vi "Compare.vi"() -> ()   [LabVIEW 2013]
panel:
  out "Test":string
  in  "Use As Reference":bool
  in  "Next":bool
  in  "pattern":string="*.png"
  out "Reference Picture":picture
  out "Test Picture":picture
  in  "Reference Directory":path=path "C:/aplot/tests/ref"
  in  "Test Directory":path=path "C:/aplot/tests/output"
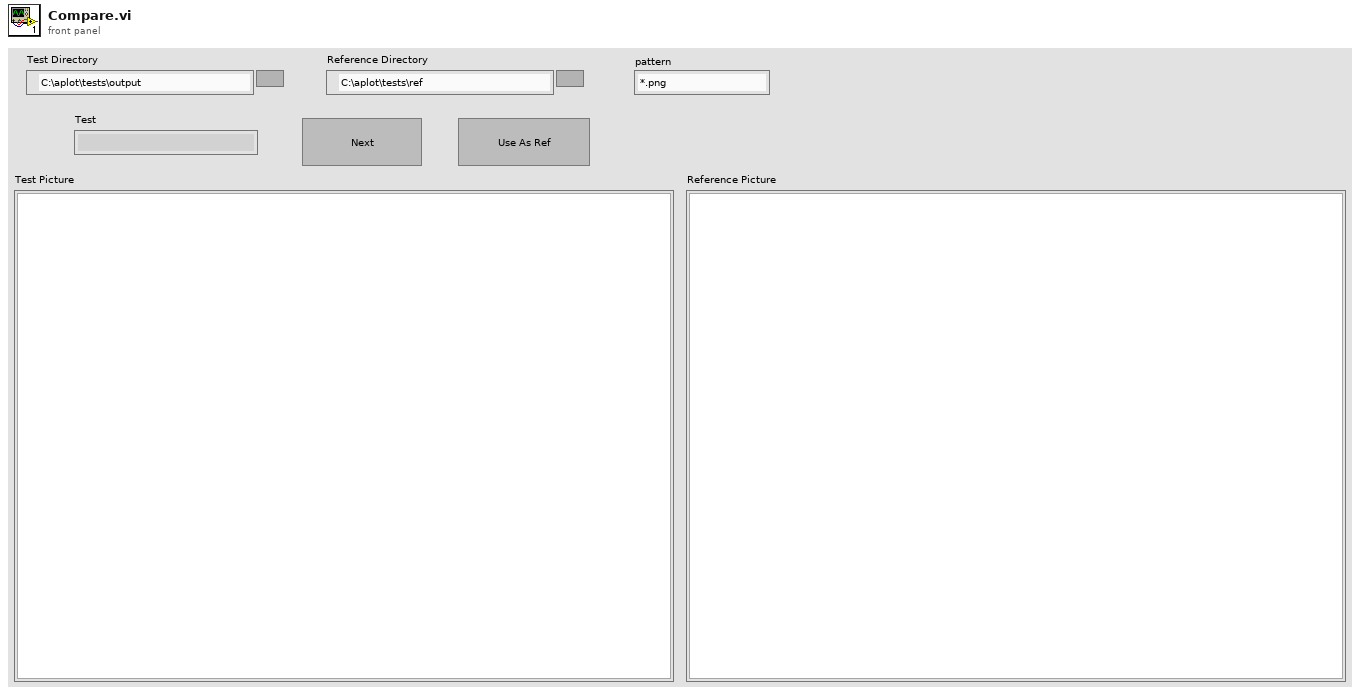
[diagram p1: front panel]
types:
  T1 = typedef "imagedata.ctl" = cluster{"image type":i32, "image depth":i32, "image":u8[], "mask":u8[], "colors":u32[], "Rectangle":cluster{"left":i16, "top":i16, "right":i16, "bottom":i16}}
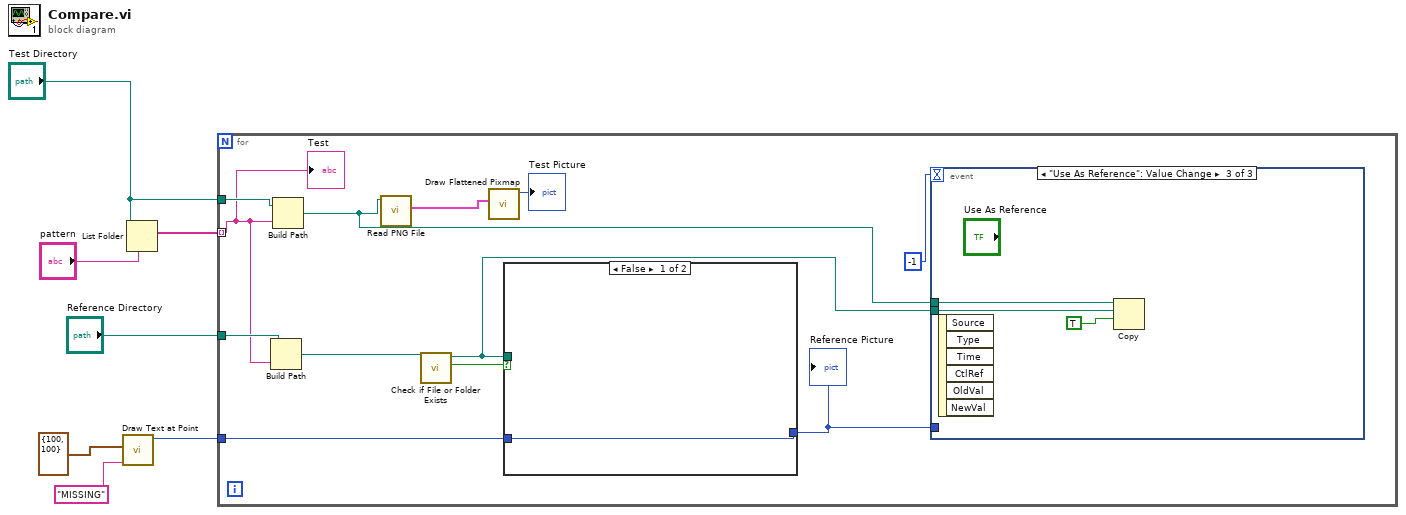
[diagram p0: block diagram]
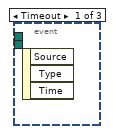
[diagram p2: hidden frame]
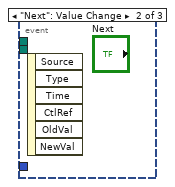
[diagram p3: hidden frame]
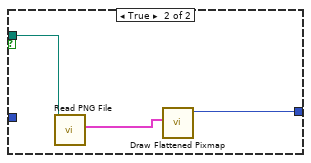
[diagram p4: hidden frame]
diagram:
  n1 = call <vilib>:"Draw Text at Point.vi"("text"="MISSING", "origin"=cluster{"x":i16, "y":i16} {"x"=100, "y"=100}) -> ("new picture"=w1:picture)  [unwired: 8 in, 1 out]
  n2 = List Folder(path="Test Directory", pattern="pattern") -> (filenames=w7:string[])  [unwired: 2 in, 3 out]
  n3 = for {
    tunnel: w7 -> [w8] mode=indexing
    tunnel: "Test Directory" -> [w19]
    tunnel: "Reference Directory" -> [w18]
    tunnel: w1 -> [w13]
    n4 = Build Path(base path=w18, name or relative path=w8) -> (appended path=w15:path)
    n5 = Build Path(base path=w19, name or relative path=w8) -> (appended path=w10:path)
    n6 = call <vilib>:"Read PNG File.vi"("path to PNG file"=w10) -> ("image data"=w17:T1)  [unwired: 8 in, 2 out]
    n7 = call <vilib>:"Check if File or Folder Exists.vi"("path"=w15) -> ("file or folder exists?"=w14:bool, "dup path"=w9:path)  [unwired: 8 in, 1 out]
    n8 = call <vilib>:"Draw Flattened Pixmap.vi"("image data"=w17) -> ("new picture"=→"Test Picture":picture)  [unwired: 8 in]
    n9 = case shown="False" w14 {
      tunnel: w9 -> [_ w25]
      tunnel: [w23 w24] -> w12
      tunnel: w13 -> [w23 _]
      frame False {
      }
      frame True {
        n10 = call <vilib>:"Read PNG File.vi"("path to PNG file"=w25) -> ("image data"=w26:T1)  [unwired: 8 in, 2 out]
        n11 = call <vilib>:"Draw Flattened Pixmap.vi"("image data"=w26) -> ("new picture"=w24:picture)  [unwired: 8 in]
      }
    }
    "Reference Picture" <- w12
    n12 = event shown="[2] \"Use As Reference\": Value Change" {
      selector: _ -> [_ _ _]
      dyn-events: _ -> [_ _ _]
      timeout: -1 -> [_ _ _]
      tunnel: w12 -> [_ _ _]
      tunnel: w10 -> [_ _ w22]
      tunnel: w9 -> [_ _ w21]
      event Timeout {
        n13 = event-data() -> ()  [unwired: 1 in, 3 out]
      }
      event "Next": Value Change {
        n14 = event-data() -> ()  [unwired: 1 in, 6 out]
      }
      event "Use As Reference": Value Change {
        n15 = event-data() -> ()  [unwired: 1 in, 6 out]
        n16 = Copy(9:TRUE ("overwrite (F)"), 10:w21, 11:w22) -> ()  [unwired: 2 in, 3 out]
      }
    }
    "Test" <- w8
  }
